vi "Check Loop Error.vi"(4 "Ignore Errors":i32[](array[numeric]), 6 "Log-Only Errors":i32[](array[numeric]), 9 "Critical Errors":i32[](array[numeric]), 10 "error to process":errorcluster, 11 "Message Queue":refnum<queue>) -> (2 "Enqueued Error?":bool, 3 "dup Message Queue":refnum<queue>)   [LabVIEW 2017]
uses:
  Message Queue/Message Cluster.ctl
  controls/Error Type.ctl
  Message Queue/Message Queue.lvlib
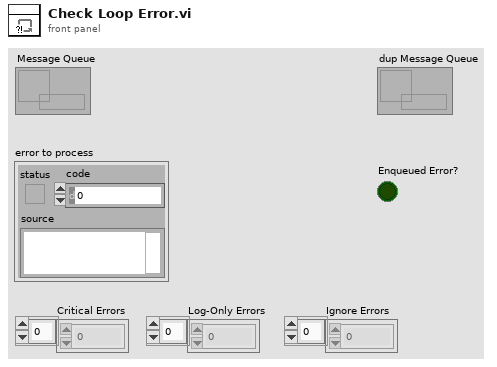
[diagram p1: front panel]
types:
  T1 = typedef "Error Type.ctl" = enum16{"Log-Only Error", "Non-Critical Error", "Critical Error"}
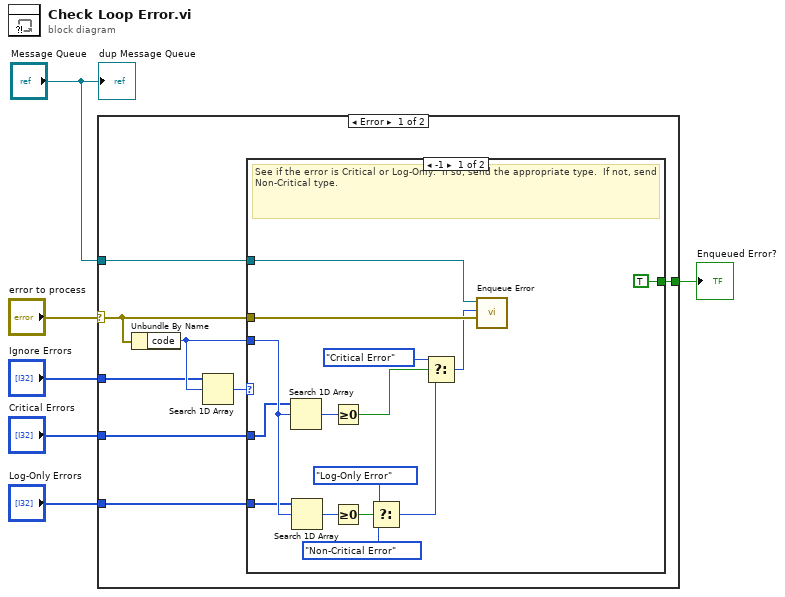
[diagram p0: block diagram]
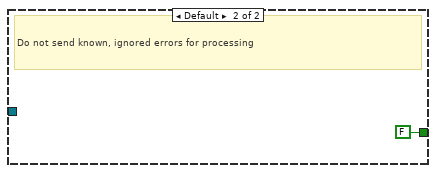
[diagram p2: hidden frame]
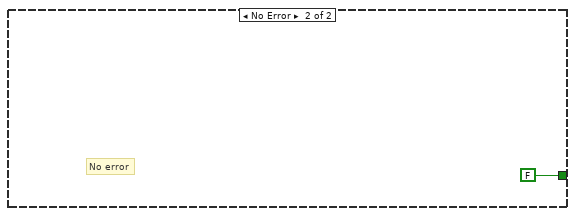
[diagram p3: hidden frame]
diagram:
  n1 = case shown="Error" "error to process" {
    selector: "error to process" -> [w11 _]
    tunnel: "Message Queue" -> [w14 _]
    tunnel: "Ignore Errors" -> [w10 _]
    tunnel: "Critical Errors" -> [w9 _]
    tunnel: "Log-Only Errors" -> [w8 _]
    tunnel: [w7 FALSE] -> w1
    frame Error {
      n2 = Unbundle By Name(w11) -> ("code"=w12:i32)
      n3 = Search 1D Array(1D array=w10, element=w12) -> (index of element=w13:i32)  [unwired: 1 in]
      n4 = case shown="-1" w13 {
        tunnel: w11 -> [w28 _]
        tunnel: w14 -> [w29 _]
        tunnel: w12 -> [w27 _]
        tunnel: w9 -> [w17 _]
        tunnel: w8 -> [w16 _]
        tunnel: [TRUE FALSE] -> w7
        frame -1 {
          # "See if the error is Critical or Log-Only.  If so, send the appropriate type.  If not, send Non-Critical type."
          n5 = Search 1D Array(1D array=w17, element=w27) -> (index of element=w26:i32)  [unwired: 1 in]
          n6 = Search 1D Array(1D array=w16, element=w27) -> (index of element=w25:i32)  [unwired: 1 in]
          n7 = Greater Or Equal To 0?(x=w26) -> (x >= 0?=w24:bool)
          n8 = Greater Or Equal To 0?(x=w25) -> (x >= 0?=w21:bool)
          n9 = Select(t=Error_Type."Log-Only Error" ("Error Type (Non-Critical)"), s=w21, f=Error_Type."Non-Critical Error" ("Error Type (Non-Critical)")) -> (s? t:f=w19:T1)
          n10 = Select(t=Error_Type."Critical Error" ("Error Type (Non-Critical)"), s=w24, f=w19) -> (s? t:f=w22:T1)
          n11 = call "Enqueue Error.vi"("error to process"=w28, "Error Type (Non-Critical)"=w22, "Message Queue"=w29) -> ()  [unwired: 9 in]
        }
        frame Default {
          # "Do not send known, ignored errors for processing"
        }
      }
    }
    frame No Error {
      # "No error"
    }
  }
  "Enqueued Error?" <- w1
  "dup Message Queue" <- "Message Queue"
